vi "Sample--ReadData.vi"() -> ()   [LabVIEW 2013]
doc: "This samples demonstrates how to sample a finite waveform."
panel:
  out "error out":errorcluster
  in  "stop":bool
  in  "Interval(ms)":u32=10
  in  "Offset(point)":i32
  in  "Data Type":i32(ring)=2 items=["U8", "U16", "DBL"]
  in  "File Path":path=path "C:/Users/Administrator/Desktop/1.PCI"
  out "waveform":dbl[][](graph)=[[3.10546875, 3.10546875, 3.1103515625, 3.1097412109375, 3.1060791015625, 3.11279296875, 3.1097412109375, 3.1121826171875, 3.116455078125, 3.11767578125, 3.121337890625, 3.1219482421875, 3.1243896484375, 3.123779296875, 3.125, 3.1231689453125, 3.1280517578125, 3.1292724609375, 3.131103515625, 3.134765625, 3.1353759765625, 3.1353759765625, 3.1402587890625, 3.14208984375, 3.1427001953125, 3.1427001953125, 3.1475830078125, 3.1463623046875, 3.150634765625, 3.1488037109375, 3.1524658203125, 3.15185546875, 3.155517578125, 3.1585693359375, 3.15673828125, 3.157958984375, 3.162841796875, 3.162841796875, 3.1640625, 3.1671142578125, 3.167724609375, 3.1689453125, 3.170166015625, 3.1683349609375, 3.175048828125, 3.1573486328125, 3.1597900390625, 3.157958984375, 3.1591796875, 3.1549072265625, 3.15673828125, 3.1524658203125, 3.1524658203125, 3.1475830078125, 3.1494140625, 3.140869140625, 3.143310546875, 3.1396484375, 3.1390380859375, 3.13720703125, 3.13720703125, 3.1341552734375, 3.1353759765625, 3.1329345703125, 3.13232421875, 3.128662109375, 3.1268310546875, 3.1201171875, 3.125, 3.118896484375, 3.1182861328125, 3.1170654296875, 3.1201171875, 3.1158447265625, 3.114013671875, 3.1085205078125, 3.1097412109375, 3.1060791015625, 3.1097412109375, 3.1011962890625, 3.1036376953125, 3.0999755859375, 3.1005859375, 3.09814453125, 3.0963134765625, 3.09326171875, 3.094482421875, 3.0859375, 3.0908203125, 3.08837890625, 3.0865478515625, 3.084716796875, 3.084716796875, 3.0804443359375, 3.0804443359375, 3.07373046875, 3.0780029296875, 3.07373046875, 3.074951171875, 3.0706787109375, 3.0706787109375, 3.0657958984375, 3.067626953125, 3.065185546875, 3.0645751953125, 3.0596923828125, 3.062744140625, 3.060302734375, 3.0548095703125, 3.0523681640625, 3.0535888671875, 3.04931640625, 3.0499267578125, 3.046875, 3.046875, 3.0438232421875, 3.0426025390625, 3.0438232421875, 3.040771484375, 3.0377197265625, 3.035888671875, 3.033447265625, 3.031005859375, 3.028564453125, 3.0291748046875, 3.0279541015625, 3.0291748046875, 3.0218505859375, 3.0230712890625, 3.021240234375, 3.018798828125, 3.018798828125, 3.016357421875, 3.0157470703125, 3.011474609375, 3.01025390625, 3.0084228515625, 3.009033203125, 3.0059814453125, 3.001708984375, 3.004150390625, 2.9974365234375, 3.0010986328125, 2.99560546875, 2.9962158203125, 2.994384765625, 2.9937744140625, 2.9931640625, 2.9913330078125, 2.98828125, 2.9876708984375, 2.984619140625, 2.9833984375, 2.98095703125, 2.9791259765625, 2.9791259765625, 2.9791259765625, 2.9730224609375, 2.9754638671875, 2.9736328125, 2.9681396484375, 2.9681396484375, 2.9632568359375, 2.9632568359375, 2.9638671875, 2.960205078125, 2.957763671875, 2.9559326171875, 2.958984375, 2.95654296875, 2.9522705078125, 2.94921875, 2.947998046875, 2.945556640625, 2.94677734375, 2.94677734375, 2.9388427734375, 2.9400634765625, 2.9400634765625, 2.9388427734375, 2.9376220703125, 2.9345703125, 2.9327392578125, 2.9327392578125, 2.930908203125, 2.92724609375, 2.926025390625, 2.9217529296875, 2.9217529296875, 2.918701171875, 2.9217529296875, 2.9168701171875, 2.9144287109375, 2.916259765625, 2.91015625, 2.9095458984375, 2.906494140625, 2.9058837890625, 2.90283203125, 2.904052734375, 2.9034423828125, 2.899169921875, 2.899169921875, 2.8973388671875, 2.8961181640625, 2.89306640625, 2.891845703125, 2.890625, 2.889404296875, 2.8887939453125, 2.8851318359375, 2.8851318359375, 2.8814697265625, 2.879638671875, 2.8790283203125, 2.8759765625, 2.8729248046875, 2.874755859375, 2.872314453125, 2.87353515625, 2.8662109375, 2.8656005859375, 2.8668212890625, 2.8656005859375, 2.8607177734375, 2.861328125, 2.8594970703125, 2.8582763671875, 2.8521728515625, 2.8509521484375, 2.850341796875, 2.84912109375, 2.8485107421875, 2.8466796875, 2.8448486328125, 2.8448486328125, 2.841796875, 2.8399658203125, 2.838134765625, 2.8387451171875, 2.833251953125, 2.8314208984375, 2.8326416015625, 2.82958984375, 2.82470703125, 2.82470703125, 2.82470703125, 2.8228759765625, 2.822265625, 2.81982421875, 2.816162109375, 2.8179931640625, 2.8131103515625, 2.8192138671875, 2.81005859375, 2.808837890625, 2.8076171875, 2.806396484375, 2.8033447265625, 2.80517578125, 2.8009033203125, 2.80029296875, 2.796630859375, 2.7960205078125, 2.794189453125, 2.79296875, 2.791748046875, 2.7911376953125, 2.7862548828125, 2.786865234375, 2.78076171875, 2.781982421875, 2.7801513671875, 2.779541015625, 2.777099609375, 2.777099609375, 2.7740478515625, 2.774658203125, 2.769775390625, 2.76611328125, 2.7679443359375, 2.76611328125, 2.7618408203125, 2.7630615234375, 2.7606201171875, 2.7587890625, 2.757568359375, 2.7557373046875, 2.7520751953125, 2.755126953125, 2.747802734375, 2.750244140625, 2.74658203125, 2.7435302734375, 2.7435302734375, 2.7423095703125, 2.7410888671875, 2.744140625, 2.7349853515625, 2.73681640625, 2.73193359375, 2.73193359375, 2.730712890625, 2.72705078125, 2.7276611328125, 2.7252197265625, 2.7227783203125, 2.7239990234375, 2.7178955078125, 2.718505859375, 2.7154541015625, 2.713623046875, 2.7142333984375, 2.7142333984375, 2.7099609375, 2.7099609375, 2.706298828125, 2.7056884765625, 2.7056884765625, 2.703857421875, 2.7001953125, 2.6995849609375, 2.6971435546875, 2.696533203125, 2.6922607421875, 2.6934814453125, 2.6904296875, 2.689208984375, 2.6873779296875, 2.6837158203125, 2.6812744140625, 2.681884765625, 2.6800537109375, 2.67822265625, 2.67578125, 2.6739501953125, 2.672119140625, 2.67333984375, 2.6702880859375, 2.6708984375, 2.667236328125, 2.664794921875, 2.6641845703125, 2.6629638671875, 2.662353515625, 2.65869140625, 2.6556396484375, 2.6568603515625, 2.6544189453125, 2.655029296875, 2.6507568359375, 2.6483154296875, 2.645263671875, 2.6446533203125, 2.6422119140625, 2.6434326171875, 2.6416015625, 2.63671875, 2.635498046875, 2.6348876953125, 2.6348876953125, 2.6318359375, 2.6324462890625, 2.6287841796875, 2.628173828125, 2.6275634765625, 2.6251220703125, 2.62451171875, 2.6214599609375, 2.61962890625, 2.6171875, 2.6153564453125, 2.6116943359375, 2.6123046875, 2.60986328125, 2.6092529296875, 2.606201171875, 2.60498046875, 2.6031494140625, 2.603759765625, 2.5994873046875, 2.59765625, 2.5958251953125, 2.59521484375, 2.5927734375, 2.5921630859375, 2.5897216796875, 2.5927734375, 2.5872802734375, 2.587890625, 2.5836181640625, 2.5848388671875, 2.5811767578125, 2.579345703125, 2.576904296875, 2.5762939453125, 2.5738525390625, 2.574462890625, 2.5689697265625, 2.5701904296875, 2.5665283203125, 2.5640869140625, 2.5634765625, 2.5628662109375, 2.559814453125, 2.559814453125, 2.55615234375, 2.55859375, 2.5537109375, 2.554931640625, 2.552490234375, 2.5457763671875, 2.54638671875, 2.547607421875, 2.5457763671875, 2.545166015625, 2.5408935546875, 2.5384521484375, 2.5390625, 2.5347900390625, 2.5347900390625, 2.5311279296875, 2.528076171875, 2.5274658203125, 2.52685546875, 2.5244140625, 2.5213623046875, 2.520751953125, 2.5201416015625, 2.520751953125, 2.51708984375, 2.518310546875, 2.515869140625, 2.5115966796875, 2.5115966796875, 2.5103759765625, 2.506103515625, 2.506103515625, 2.5042724609375, 2.50244140625, 2.4993896484375, 2.4993896484375, 2.4981689453125, 2.49755859375, 2.4932861328125, 2.493896484375, 2.49267578125, 2.4896240234375, 2.48779296875, 2.4847412109375, 2.4847412109375, 2.481689453125, 2.481689453125, 2.4761962890625, 2.4774169921875, 2.476806640625, 2.474365234375, 2.4725341796875, 2.470703125, 2.4700927734375, 2.467041015625, 2.464599609375, 2.4627685546875, 2.46337890625, 2.4609375, 2.4591064453125, 2.4578857421875, 2.454833984375, 2.4542236328125, 2.45361328125, 2.4530029296875, 2.4505615234375, 2.4493408203125, 2.4468994140625, 2.4432373046875, 2.4420166015625, 2.4407958984375, 2.4383544921875, 2.4365234375, 2.435302734375, 2.435302734375, 2.4334716796875, 2.4322509765625, 2.4310302734375, 2.4298095703125, 2.425537109375, 2.4237060546875, 2.4224853515625, 2.4212646484375, 2.4169921875, 2.4163818359375, 2.415771484375, 2.41455078125, 2.4114990234375, 2.410888671875, 2.4090576171875, 2.4066162109375, 2.4066162109375, 2.4041748046875, 2.4017333984375, 2.401123046875, 2.398681640625, 2.3968505859375, 2.3968505859375, 2.3931884765625, 2.391357421875, 2.391357421875, 2.3870849609375, 2.3870849609375, 2.3846435546875, 2.3822021484375, 2.3822021484375]]
  in  "ReadLength\n(point)":i32=1000
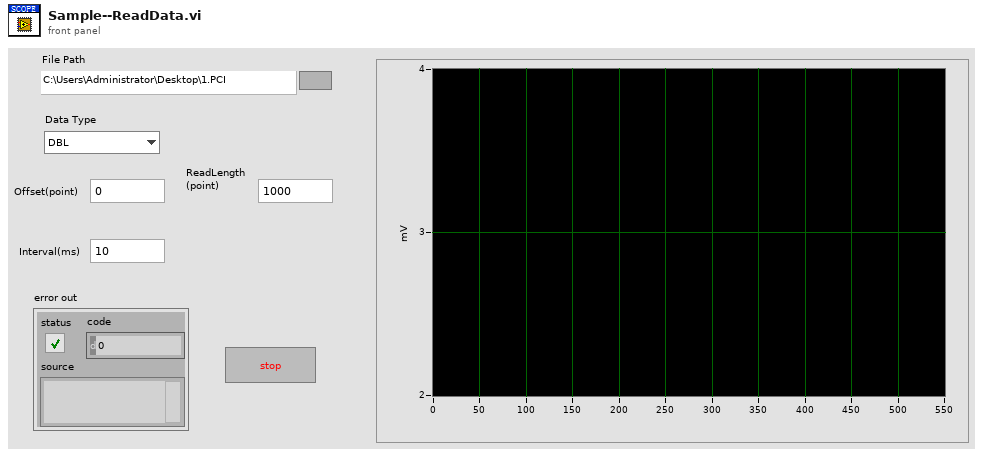
[diagram p1: front panel]
types:
  T1 = enum16{"big-endian, network order", "native, host order", "little-endian"}
  T2 = enum16{"open", "replace", "create", "open or create", "replace or create", "replace or create with confirmation"}
  T3 = cluster{"fLsbs":cluster{dbl, dbl, dbl, dbl, dbl, dbl, dbl, dbl}, "RangeValue":cluster{dbl, dbl, dbl, dbl, dbl, dbl, dbl, dbl}, "wMaxLSB":u32, "TriggerMode":i32, "actualSamples":u32, "pAvailSampsPoints":u32, "channelCount":i32}
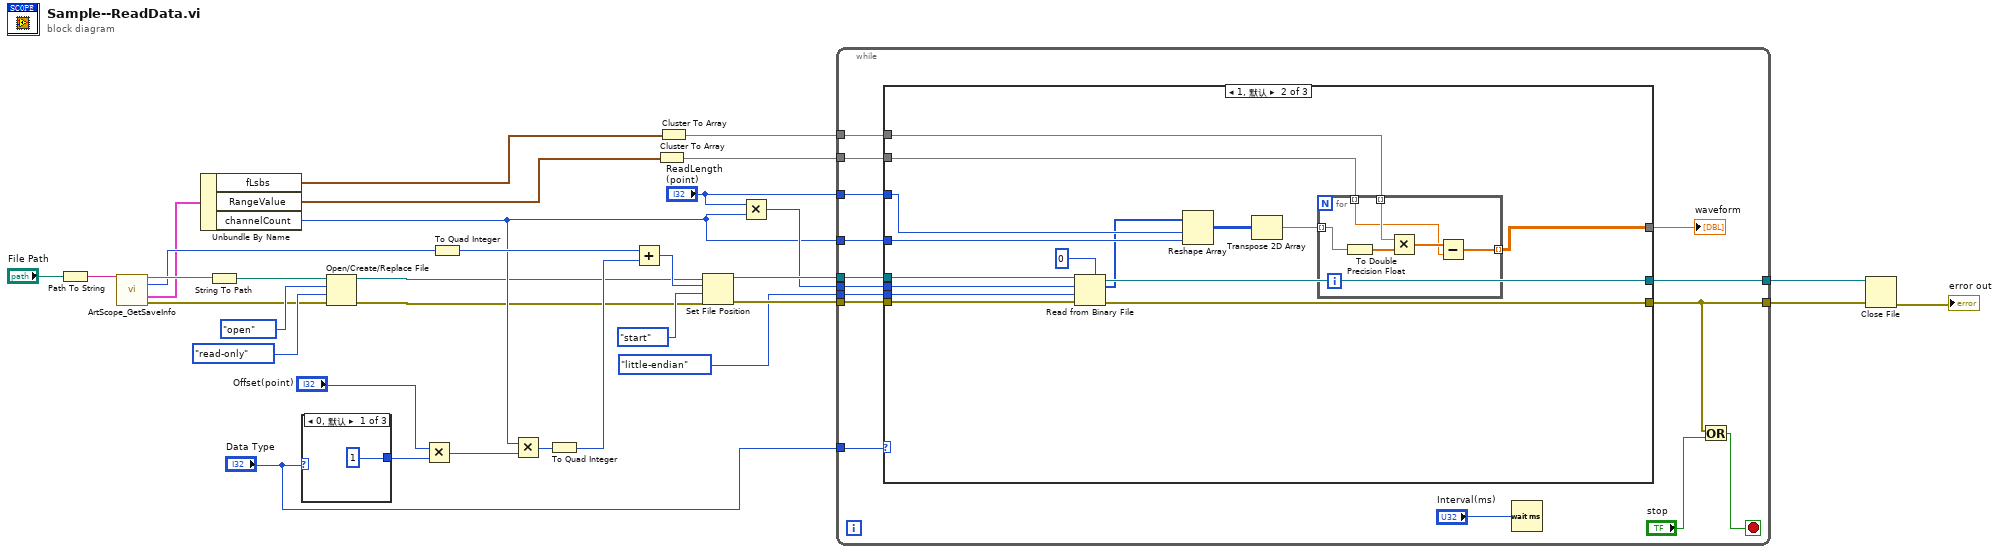
[diagram p0: block diagram]
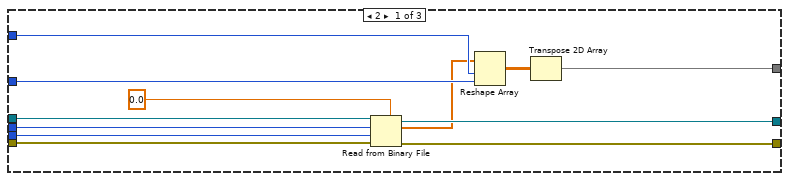
[diagram p2: hidden frame]
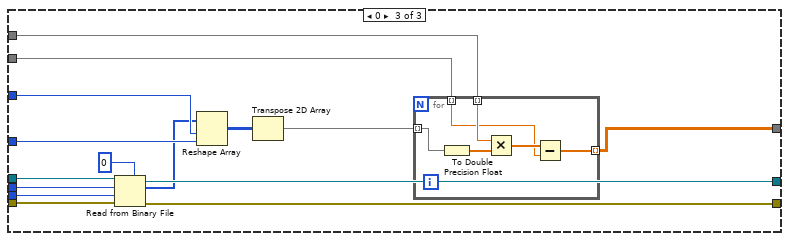
[diagram p3: hidden frame]
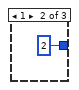
[diagram p4: hidden frame]
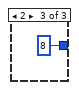
[diagram p5: hidden frame]
diagram:
  n1 = Path To String(path="File Path") -> (string=w14:string)
  n2 = call <userlib>:"ArtScope_GetSaveInfo.vi"("file name"=w14) -> ("file name"=w29:string, "header size"=w28:i32, "file wfm info"=w24:T3, "error out"=w31:errorcluster)  [unwired: 11 in]
  n3 = Unbundle By Name(w24) -> ("fLsbs"=w18:cluster{dbl, dbl, dbl, dbl, dbl, dbl, dbl, dbl}, "RangeValue"=w16:cluster{dbl, dbl, dbl, dbl, dbl, dbl, dbl, dbl}, "channelCount"=w8:i32)
  n4 = String To Path(string=w29) -> (path=w30:path)
  n5 = case shown="0, 默认" "Data Type" {
    tunnel: [1 2 8] -> w11
    frame 0, Default {
    }
    frame 1 {
    }
    frame 2 {
    }
  }
  n6 = Open/Create/Replace File(file path (use dialog)=w30, error in=w31, operation (0:open)=T2."open" ("操作(0:open)"), access (0:read/write)=enum16{"read/write", "read-only", "write-only"}."read-only" ("权限(0:read/write)")) -> (refnum out=w3:refnum<file>, error out=w2:errorcluster)  [unwired: 2 in, 1 out]
  n7 = Multiply(x="Offset(point)", y=w11) -> (x*y=w9:i32)
  n8 = To Quad Integer(1:w28) -> (0:w12:i64)
  n9 = Multiply(x=w8, y=w9) -> (x*y=w7:i32)
  n10 = To Quad Integer(1:w7) -> (0:w6:i64)
  n11 = Add(x=w12, y=w6) -> (x+y=w5:i64)
  n12 = Cluster To Array(cluster=w16) -> (array=w15:dbl[])
  n13 = Cluster To Array(cluster=w18) -> (array=w17:dbl[])
  n14 = Set File Position(offset (in bytes) (0)=w5, refnum=w3, from (0:start)=enum16{"start", "end", "current"}."start" ("自（0:起始）"), error in=w2) -> (refnum out=w26:refnum<file>, error out=w25:errorcluster)
  n15 = Multiply(x="ReadLength\n(point)", y=w8) -> (x*y=w23:i32)
  n16 = while {
    tunnel: w26 -> [w51]
    tunnel: w25 -> [w50]
    tunnel: w23 -> [w49]
    tunnel: T1."little-endian" ("字节顺序(0:big-endian, network order)") -> [w48]
    tunnel: "ReadLength\n(point)" -> [w47]
    tunnel: [w39] -> w20
    tunnel: [w46] -> w19
    tunnel: w17 -> [w45]
    tunnel: w15 -> [w44]
    tunnel: w8 -> [w43]
    tunnel: "Data Type" -> [w42]
    stop <- w37 stop-if-true
    n17 = case shown="1, 默认" w42 {
      tunnel: w51 -> [w63 w64 w99]
      tunnel: w50 -> [w62 w65 w98]
      tunnel: w49 -> [w61 w78 w97]
      tunnel: w48 -> [w60 w77 w96]
      tunnel: w47 -> [w59 w76 w95]
      tunnel: w43 -> [w58 w75 w94]
      tunnel: [w56 w66 w85] -> w41
      tunnel: [w55 w73 w92] -> w39
      tunnel: [w54 w72 w91] -> w46
      tunnel: w45 -> [_ w68 w87]
      tunnel: w44 -> [_ w67 w86]
      frame 2 {
        n18 = Read from Binary File(5:0.0, 8:w62, 9:w60, 10:w61, 11:w63) -> (0:w55:errorcluster, 2:w52:dbl[], 3:w54:refnum<file>)  [unwired: 1 in, 1 out]
        n19 = Reshape Array(w52, w59, w58) -> (w57:dbl[][])
        n20 = Transpose 2D Array(2D array=w57) -> (transposed array=w56:dbl[][])
      }
      frame 1, Default {
        n21 = Read from Binary File(5:u16 0, 8:w65, 9:w77, 10:w78, 11:w64) -> (0:w73:errorcluster, 2:w70:u16[], 3:w72:refnum<file>)  [unwired: 1 in, 1 out]
        n22 = Reshape Array(w70, w76, w75) -> (w74:u16[][])
        n23 = Transpose 2D Array(2D array=w74) -> (transposed array=w69:u16[][])
        n24 = for {
          tunnel: w69 -> [w79] mode=indexing
          tunnel: w67 -> [w81] mode=indexing
          tunnel: w68 -> [w84] mode=indexing
          tunnel: [w80] -> w66 mode=indexing
          n25 = To Double Precision Float(number=w79) -> (double precision float=w83:dbl[])
          n26 = Multiply(x=w84, y=w83) -> (x*y=w82:dbl[])
          n27 = Subtract(x=w82, y=w81) -> (x-y=w80:dbl[])
        }
      }
      frame 0 {
        n28 = Read from Binary File(5:u8 0, 8:w98, 9:w96, 10:w97, 11:w99) -> (0:w92:errorcluster, 2:w89:u8[], 3:w91:refnum<file>)  [unwired: 1 in, 1 out]
        n29 = Reshape Array(w89, w95, w94) -> (w93:u8[][])
        n30 = Transpose 2D Array(2D array=w93) -> (transposed array=w88:u8[][])
        n31 = for {
          tunnel: w88 -> [w100] mode=indexing
          tunnel: w86 -> [w102] mode=indexing
          tunnel: w87 -> [w105] mode=indexing
          tunnel: [w101] -> w85 mode=indexing
          n32 = To Double Precision Float(number=w100) -> (double precision float=w104:dbl[])
          n33 = Multiply(x=w105, y=w104) -> (x*y=w103:dbl[])
          n34 = Subtract(x=w103, y=w102) -> (x-y=w101:dbl[])
        }
      }
    }
    "waveform" <- w41
    n35 = Wait (ms)(milliseconds to wait="Interval(ms)") -> ()  [unwired: 1 out]
    n36 = Or(x=w39, y="stop") -> (x .or. y?=w37:bool)
  }
  n37 = Close File(refnum=w19, error in=w20) -> (error out=→"error out":errorcluster)  [unwired: 1 out]
